vi "OCR_Determine Color and Text.vi"(8 "Error":errorcluster, 11 "Border Removed":T3) -> (0 "Error Out":errorcluster, 1 "Colors Out":T1, 2 "Text Out":T4[](array[typedef]), 3 "Header Out":bool, 4 "Status Of Each Line Out":bool[](array[boolean]))   [LabVIEW 2009]
uses:
  Controls/String_Picture/STRING_Line Display.ctl
  Controls/Array/Color Box Array_2D Icon Viewer.ctl
  Controls/Cluster/Cluster_Icon Color Set.ctl
  Controls/Enum/ENUM_Frame Template Select.ctl
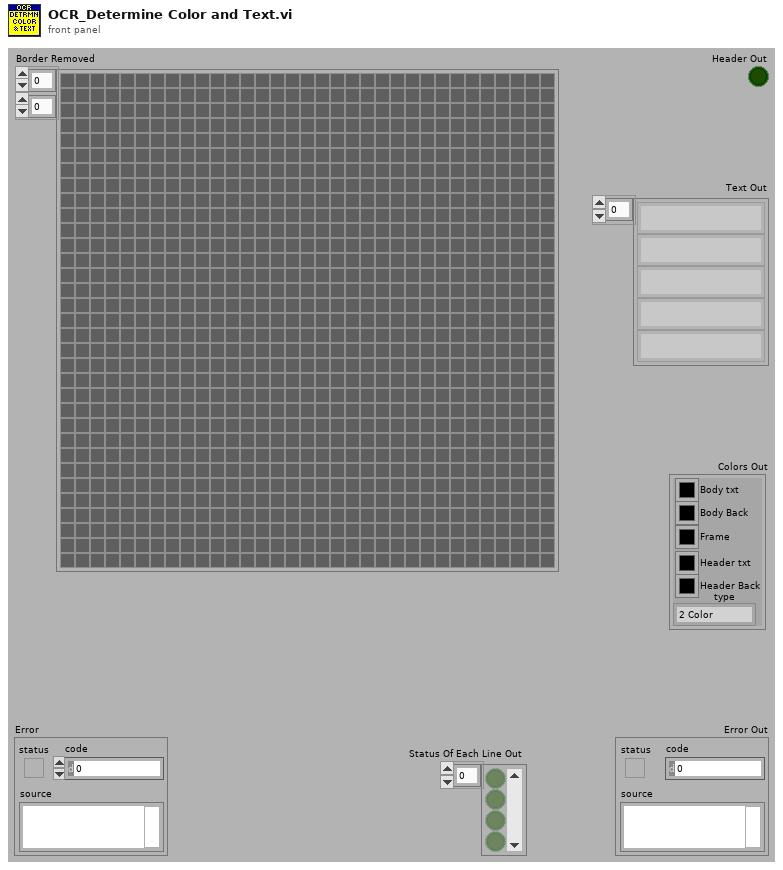
[diagram p1: front panel]
types:
  T1 = typedef "Cluster_Icon Color Set.ctl" = cluster{"Body txt":u32, "Body Back":u32, "Frame":u32, "Header txt":u32, "Header Back":u32, "type":T2}
  T2 = typedef "ENUM_Frame Template Select.ctl" = enum16{"2 Color", "5 Color"}
  T3 = typedef "Color Box Array_2D Icon Viewer.ctl" = u32[][]
  T4 = typedef "STRING_Line Display.ctl" = string
  T5 = typedef "Cluster_Text Color Set.ctl" = cluster{"BG":u32, "FG":u32}
  T6 = typedef "ENUM_Line Letter Type.ctl" = enum16{"Unknown", "Letter", "Seperator", "Seperator or Letter"}
  T7 = typedef "Cluster_Line Location and status.ctl" = cluster{"Index":i16[], "Status":bool[], "Size":i32[]}
  T8 = typedef "Cluster_Text Rect.ctl" = cluster{"window":T9, "Color":T5, "Status":bool}
  T9 = typedef "Cluster_Region info.ctl" = cluster{"Left":i32, "Top":i32, "Right":i32, "Bottom":i32, "Width":u32, "Height":u32, "Start":T10}
  T10 = typedef "Cluster_Top Left position.ctl" = cluster{"Left":i32, "Top":i32}
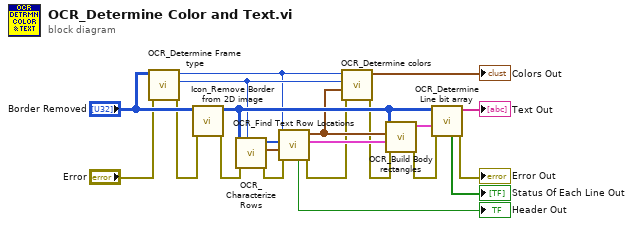
[diagram p0: block diagram]
diagram:
  n1 = call "OCR_Determine Frame type.vi"("Error"="Error", "2D Image"="Border Removed") -> ("Error Out"=w12:errorcluster, "Frame Out"=w8:T2, "Border Color Out"=w1:u32)  [unwired: 7 in]
  n2 = call "Icon_Remove Border from 2D image.vi"("Error"=w12, "2D Image"="Border Removed") -> ("Error Out"=w15:errorcluster, "Border Removed Out"=w16:T3)  [unwired: 8 in]
  n3 = call "OCR_Characterize Rows.vi"("Frame"=w8, "Error"=w15, "2D Image"=w16) -> ("Error Out"=w18:errorcluster, "Top Color Array Out"=w17:T5[], "Row Type Out"=w2:T6[])  [unwired: 6 in]
  n4 = call "OCR_Find Text Row Locations.vi"("Error"=w18, "Color Array"=w17, "Row Type Array"=w2, "Frame Color"=w1) -> ("Error Out"=w6:errorcluster, "Body Cluster Out"=w20:T7, "Color Array Out"=w10:T5[], "Header Out"=→"Header Out":bool)  [unwired: 3 in, 1 out]
  n5 = call "OCR_Determine colors.vi"("Error"=w6, "Color Array"=w10, "Frame Type"=w8, "Border Color"=w1) -> ("Error Out"=w5:errorcluster, "Colors Out"=→"Colors Out":T1)  [unwired: 6 in]
  n6 = call "OCR_Build Body rectangles.vi"("Error"=w5, "Text Location"=w20, "Color Array"=w10, "2D Image"=w16) -> ("Error Out"=w21:errorcluster, "Body Rect Array Out"=w19:T8[])  [unwired: 6 in]
  n7 = call "OCR_Determine Line bit array.vi"("Error"=w21, "Body Rect Array"=w19, "Border Removed"=w16) -> ("Error Out"=→"Error Out":errorcluster, "Text Out"=→"Text Out":T4[], "Status Of Each Line Out"=→"Status Of Each Line Out":bool[])  [unwired: 6 in]
